vi "CloseConnectionWithDevice.vi"(8 "error in (no error)":errorcluster) -> (0 "error out":errorcluster)   [LabVIEW 2023, in "DeviceManager.lvlib"]
uses:
  DeviceManager.lvlib
panel:
  # "Connector Pane"
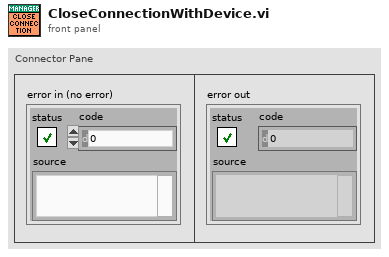
[diagram p1: front panel]
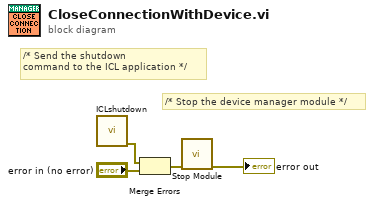
[diagram p0: block diagram]
diagram:
  # "/* Stop the device manager module */"
  # "/* Send the shutdown\ncommand to the ICL application */"
  n1 = call "ICLshutdown.vi"() -> ("error out"=w4:errorcluster)  [unwired: 11 in]
  n2 = Merge Errors(w4, "error in (no error)") -> (w2:errorcluster)
  n3 = call "Stop Module.vi"("error in"=w2) -> ("error out"=→"error out":errorcluster)  [unwired: 10 in]
